vi "Path_Test_TankRobot_ScanIndex.vi"() -> ()   [LabVIEW 2018]
uses:
  Pathfinder-Lib/VIs/Waypoint.ctl
  <vilib>/Rock Robotics/WPI/DriverStation/WPI_DriverStationRobotMode2.ctl
  Pathfinder-Lib/VIs/Wheel_Ctrl_Path_Element.ctl
  Pathfinder-Lib/VIs/Wheel_Ctrl_Path.ctl
  <vilib>/Rock Robotics/SystemInterfaces/AI/FPGA_AIGyroChannel.ctl
  <vilib>/Rock Robotics/SystemInterfaces/DIO/FPGA_DIOChannel.ctl
  <vilib>/Rock Robotics/WPI/Encoder/WPI_EncoderType.ctl
  <vilib>/Rock Robotics/SystemInterfaces/DIO/FPGA_DIOPWMChannel.ctl
  <vilib>/Rock Robotics/WPI/SafetyOutput/WPI_SafetyOutputConfigMenu.ctl
  <vilib>/Rock Robotics/WPI/Gyro/WPI_GyroAnalogOpen.vi
  <vilib>/Rock Robotics/WPI/Counter/WPI_CounterDigitalInputToDigitalSource.vi
  <vilib>/Rock Robotics/WPI/RobotDrive/WPI_RobotDriveOpen2MotorWithTalon.vi
  Robot Global Data.vi
  Secret_Control_Library_Protected/TIME_GET.vi
  <vilib>/addons/control/pid/pid.llb/PID (DBL).vi
  <vilib>/Rock Robotics/Network Tables/NT Write Numeric Array.vi
  <vilib>/Rock Robotics/Network Tables/NT Write Number.vi
  Pathfinder-Lib/Pathfinder.lvlib
  <vilib>/addons/control/pid/NI_PID_pid.lvlib
  Secret_Control_Library_Protected/Secret_Control_Library_Protected.lvlib
panel:
  out "Path \nSpeed > \nMax":bool
  in  "Stop\nProgram":bool
  out "Path Distance":dbl[](array[numeric]) format="%19.2f"
  out "Robot\nExecuting":bool
  in  "Execute\nPath":bool
  out "Ready to \nExecute":bool
  in  "Calculate\nPath":bool
  out "Heading Demand":dbl format="%18.2f"
  out "Gyro Comp":dbl format="%18.2f"
  out "Heading":dbl format="%18.2f"
  in  "Gyro Comp PID gains":T1={"proportional gain (Kc)"=0.065, "integral time (Ti, min)"=0.004, "derivative time (Td, min)"=0.0} {"derivative time (Td, min)" format="%.4f"; "integral time (Ti, min)" format="%.4f"; "proportional gain (Kc)" format="%.4f"}
  out "Path calculation error":errorcluster
  out "Distance":dbl[](array[numeric]) format="%19.2f"
  in  "Use Gyro\nCompensation":bool=TRUE
  out "Heading Error":dbl format="%14.2f"
  out "Distance Error":dbl[](array[numeric]) format="%14.2f"
  out "Robot Mode":T2
  in  "Tab Control":T3(tab)
  in  "max_velocity":dbl=51.5
  in  "max_acceleration":dbl=30.0
  in  "max_jerk":dbl=120.0
  in  "wheelbase_width":dbl=20.866
  out "Real max speed":dbl
  out "Position":cluster{dbl[], dbl[]}[](graph)
  out "Path":T4(graph)
  out "Size":i32
  out "Robot Path Data":T5[](array[typedef]) {"D Time" format="%13.3f"; "Angle" format="%13.3f"; "R dist" format="%13.3f"; "L dist" format="%13.3f"; "R spd" format="%13.3f"; "L spd" format="%13.3f"; "T Time" format="%13.3f"}
  out "Wheel dmd":T6(graph)
  out "Gyro Cht":cluster{"GyroContinuous":dbl, "Angle":dbl}(graph)
  out "Err Chart":cluster{dbl, dbl, dbl}(graph)
  in  "sample_count":i32=1000
  in  "Path Results\ndT":dbl=0.02 format="%7.3f"
  in  "?":T7[](array[typedef])=[{"x"=12.0, "y"=60.0, "angle"=0.0}, {"x"=132.0, "y"=125.0, "angle"=60.0}]
  # "PATH DEFINITION"
  # "ROBOT EXECUTION"
  # "SEC"
  # "Instructions:\nThis should run on a PC simulated robot on or a real robot that has the same motors and sensors.\n1) Enter robot data on Robot Data Tab\n2) Define your path definitions.\n3) Define the time increment.  0.020 is chosen since that matches the normal loop time.\n4) Press calculate path.  If a good path was calculated it will be displayed on the Tank Data tab, and the Ready to Execute will indicate execution can begin.\nThe path can be recalculated many times before selecting execute.\n5) Start the FRC driver station.\n6) Press the execute path button.  This will start the robot simulation, or start running on the roboRIO depending on which target is selected.\n7) On the driver station, select Autonomous Enabled mode to start path execution.\n8) When finished, the graph tabs can be reviwed.  (Usiing the chart tabs during operation breaks the simulation.\n9) When completely done press the Stop Program button to end the programs execution.\n\nNotes:\n- This program alters the left and right motor demands during execution to attempt to match the heading angle demand.  The \nsimulated robot has a lot of drive friction when turning that affects operation.  This example does not include encoder compensation.\nThis could be added.\n- The path generation logic doesn't account distribution of speed to the left and right wheels.  As a result the maximum speed can be exceeded.\nIf this happens, but Path Speed > Max light will light and Ready to Execute will not light.  Lower the maximum speed in the Robot Data tab\nand recalulate the path."
  # "ROBOT DATA"
  # "INCHES/SEC"
  # "INCHES/SEC^2"
  # "?? INCHES/SEC^3"
  # "Simulated robot is 20.866"
  # "INCHES"
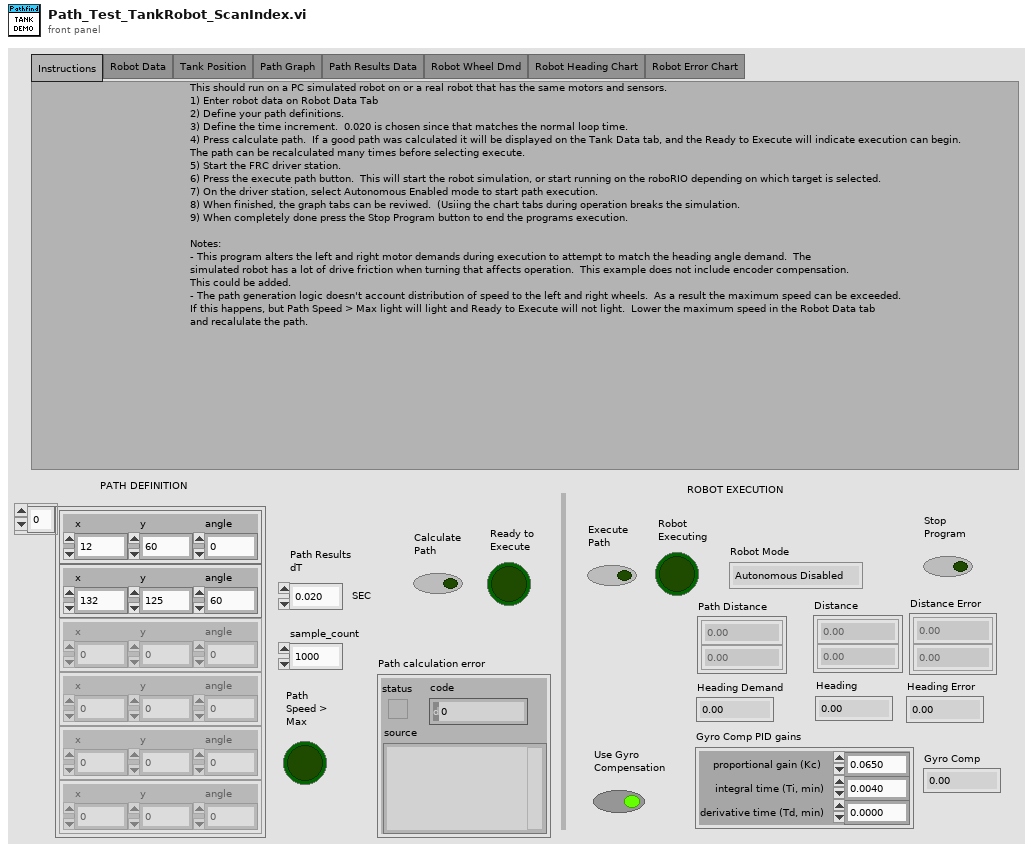
[diagram p1: front panel]
types:
  T1 = cluster{"proportional gain (Kc)":dbl, "integral time (Ti, min)":dbl, "derivative time (Td, min)":dbl}
  T2 = typedef "WPI_DriverStationRobotMode2.ctl" = enum16{"Autonomous Disabled", "Autonomous Enabled", "Teleop Disabled", "Teleop Enabled", "Disconnected", "Finish", "Test Disabled", "Test Enabled", "Emergency Stopped"}
  T3 = enum32{"Instructions", "Robot Data", "Tank Position", "Path Graph", "Path Results Data", "Robot Wheel Dmd", "Robot Heading Chart", "Robot Error Chart"}
  T4 = cluster{"position":dbl, "velocity":dbl, "acceleration":dbl, "jerk":dbl, "heading":dbl}[]
  T5 = typedef "Pathfinder.lvlib/Wheel_Ctrl_Path_Element.ctl" = cluster{"T Time":dbl, "L spd":dbl, "R spd":dbl, "L dist":dbl, "R dist":dbl, "Angle":dbl, "D Time":dbl}
  T6 = cluster{"Output":dbl, "Output":dbl, "output":dbl}
  T7 = typedef "Pathfinder.lvlib/Waypoint.ctl" = cluster{"x":dbl, "y":dbl, "angle":dbl}
  T8 = typedef "Pathfinder.lvlib/Wheel_Ctrl_Path.ctl" = cluster{"Wheel_Ctrl_Elements":T5[], "NumberOfElements":u32, "DeltaMillseconds":i32}
  T9 = typedef "Pathfinder.lvlib/Segment.ctl" = cluster{"dt":dbl, "x":dbl, "y":dbl, "position":dbl, "velocity":dbl, "acceleration":dbl, "jerk":dbl, "heading":dbl}
  T10 = cluster{"position":dbl, "velocity":dbl, "acceleration":dbl, "jerk":dbl, "heading":dbl}
  T11 = typedef "WPI_SafetyOutputConfigMenu.ctl" = enum16{"Enable", "Disable"}
  T12 = typedef "WPI_EncoderType.ctl" = enum16{"1x", "2x", "4x"}
  T13 = typedef "FPGA_AIGyroChannel.ctl" = enum8{"AI 0", "AI 1", "Invalid"}
  T14 = typedef "FPGA_DIOPWMChannel.ctl" = enum8{"PWM 0", "PWM 1", "PWM 2", "PWM 3", "PWM 4", "PWM 5", "PWM 6", "PWM 7", "PWM 8", "PWM 9", "PWM MXP 0", "PWM MXP 1", "PWM MXP 2", "PWM MXP 3", "PWM MXP 4", "PWM MXP 5", "PWM MXP 6", "PWM MXP 7", "PWM MXP 8", "PWM MXP 9", "Invalid"}
  T15 = typedef "FPGA_DIOChannel.ctl" = enum8{"DIO 0", "DIO 1", "DIO 2", "DIO 3", "DIO 4", "DIO 5", "DIO 6", "DIO 7", "DIO 8", "DIO 9", "DIO MXP 0", "DIO MXP 1", "DIO MXP 2", "DIO MXP 3", "DIO MXP 4", "DIO MXP 5", "DIO MXP 6", "DIO MXP 7", "DIO MXP 8", "DIO MXP 9", "DIO MXP 10", "DIO MXP 11", "DIO MXP 12", "DIO MXP 13", "DIO MXP 14", "DIO MXP 15", "SPI Port CS1", "SPI Port CS2", "SPI Port CS3", "SPI Port MISO", "SPI Port MOSI", "Invalid"}
  T16 = typedef "WPI_RobotDriveDevRef.ctl" = cluster{"DevStatus":errorcluster, "Motors[]":T17[], "Square Inputs":bool, "Max Output":dbl}
  T17 = typedef "WPI_MotorControlDeviceRef.ctl" = cluster{"DeviceStatus":errorcluster, "Type":T18, "PWM":cluster{"PWM Channel":T14, "DeadBand":T19}, "CAN":cluster{"Device Number":u8, "SetOutput VI Ref":variant, "GetOutput VI Ref":variant, "Enable VI Ref":variant, "Disable VI Ref":variant, "Data":variant}, "Invert":bool, "DIO PWM":cluster{"PWM \"Enable\" Channel":T14, "DIOChannel":T15, "PWM Rate":dbl}}
  T18 = typedef "WPI_MotorControlType.ctl" = enum16{"PWM", "CAN", "DIO PWM"}
  T19 = typedef "WPI_PWMDeadband.ctl" = cluster{"Name":string, "maxPositivePwm":i32, "minPositivePwm":i32, "centerPwm":i32, "maxNegativePwm":i32, "minNegativePwm":i32, "angularRange":u16}
  T20 = typedef "WPI_DigitalInputDevRef.ctl" = cluster{"DevStatus":errorcluster, "DIO Channel":T15}
  T21 = typedef "FPGA_CounterEncoderSourceConvertionLVSourceType.ctl" = cluster{"DevStatus":errorcluster, "AnalogTriggerMode?":bool, "DigitalMode":cluster{"DIO Channel":T22}, "AnalogTriggerMode":cluster{"AnalogTriggerIndex":T23, "OutputType":T24}}
  T22 = typedef "FPGA_DIODigitalSourceChannel.ctl" = enum8{"DIO 0", "DIO 1", "DIO 2", "DIO 3", "DIO 4", "DIO 5", "DIO 6", "DIO 7", "DIO 8", "DIO 9", "DIO MXP 0", "DIO MXP 1", "DIO MXP 2", "DIO MXP 3", "DIO MXP 4", "DIO MXP 5", "DIO MXP 6", "DIO MXP 7", "DIO MXP 8", "DIO MXP 9", "DIO MXP 10", "DIO MXP 11", "DIO MXP 12", "DIO MXP 13", "DIO MXP 14", "DIO MXP 15", "SPI Port CS1", "SPI Port CS2", "SPI Port CS3", "SPI Port MISO", "SPI Port MOSI", "Disabled"}
  T23 = typedef "FPGA_AnalogTriggerIndex.ctl" = enum8{"Trig 0", "Trig 1", "Trig 2", "Trig 3", "Trig 4", "Trig 5", "Trig 6", "Trig 7", "Invalid"}
  T24 = typedef "FPGA_AnalogTriggerOutType.ctl" = enum16{"InWindow", "TriggerState", "Rising", "Falling"}
  T25 = typedef "WPI_EncoderDevRef.ctl" = cluster{"DevStatus":errorcluster, "EncoderIndex":T26, "CounterIndex":T27, "DistancePerCount":dbl, "Decoding Type":T12}
  T26 = typedef "FPGA_EncoderIdx.ctl" = enum8{"Enc 0", "Enc 1", "Enc 2", "Enc 3", "Enc 4", "Enc 5", "Enc 6", "Enc 7", "Invalid"}
  T27 = typedef "FPGA_CounterCtrSystemIndex.ctl" = enum8{"Ctr 0", "Ctr 1", "Ctr 2", "Ctr 3", "Ctr 4", "Ctr 5", "Ctr 6", "Ctr 7", "Invalid"}
  T28 = typedef "WPI_GyroDevRef.ctl" = cluster{"DevStatus":errorcluster, "Analog Channel":T29, "Gain (VoltsPerDegree/Second)":dbl, "Gyro Type":enum16{"Analog", "XRS450"}, "Handle":i32, "SPI Bus":T30, "Device Found":bool, "Sample Rate":dbl, "Calibrate On Open":bool, "Offset":dbl}
  T29 = typedef "FPGA_AIChannel.ctl" = enum8{"AI 0", "AI 1", "AI 2", "AI 3", "AI MXP 0", "AI MXP 1", "AI MXP 2", "AI MXP 3", "Invalid"}
  T30 = typedef "spi_bus.ctl" = enum16{"SPI On-Board, CS0", "SPI On-Board, CS1", "SPI On-Board, CS2", "SPI On-Board, CS3", "SPI MXP", "Invalid"}
  T31 = cluster{"GyroContinuous":dbl, "GyroContinuous":dbl}
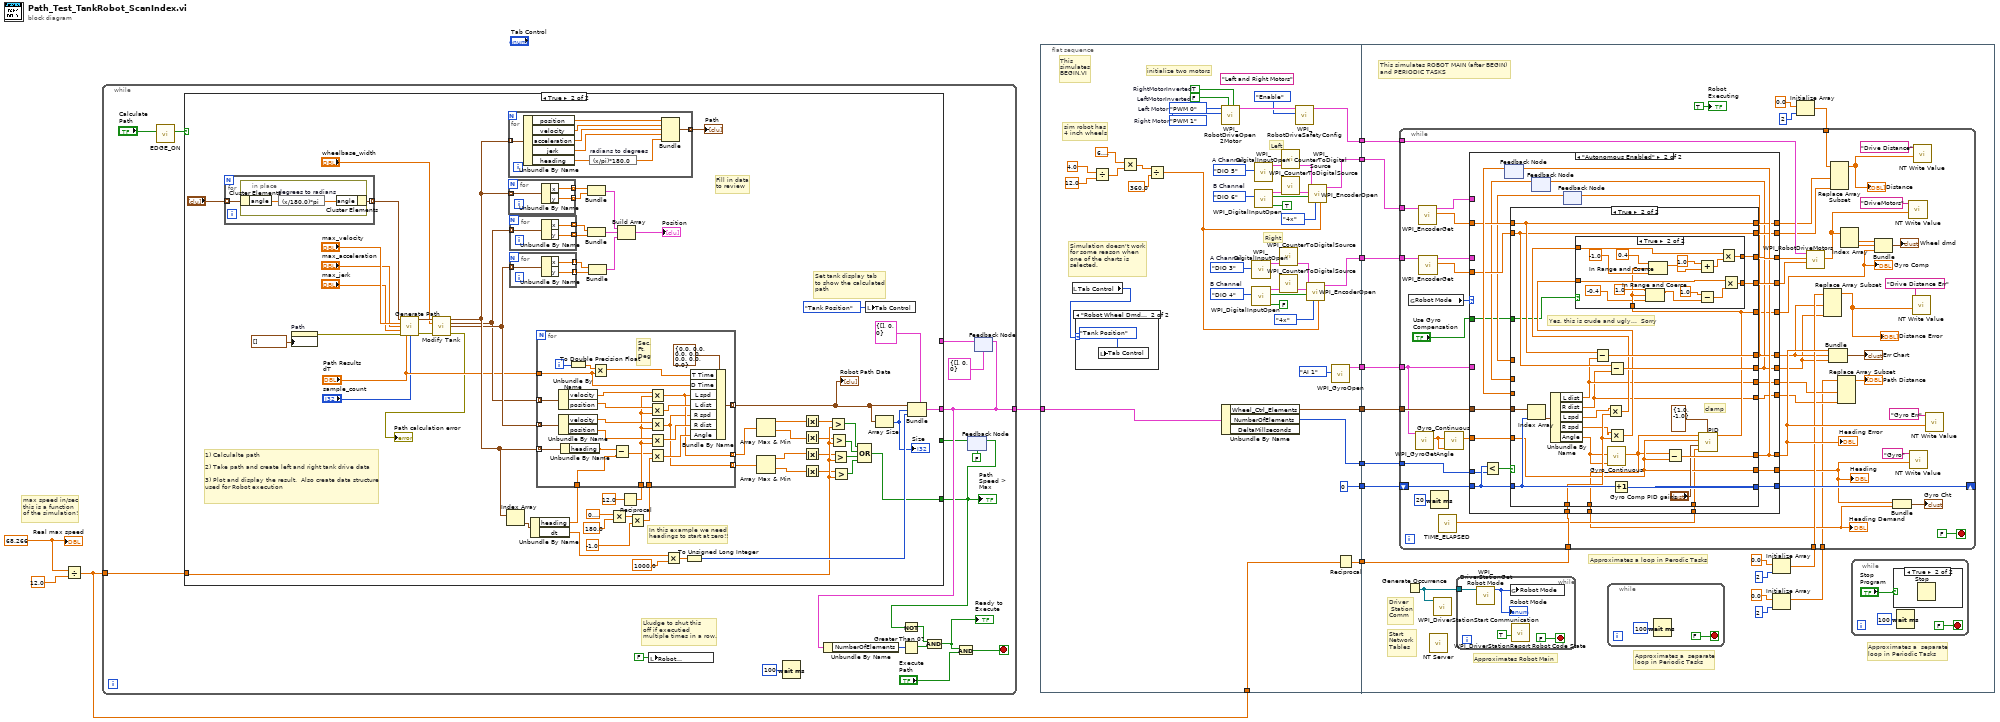
[diagram p0: block diagram]
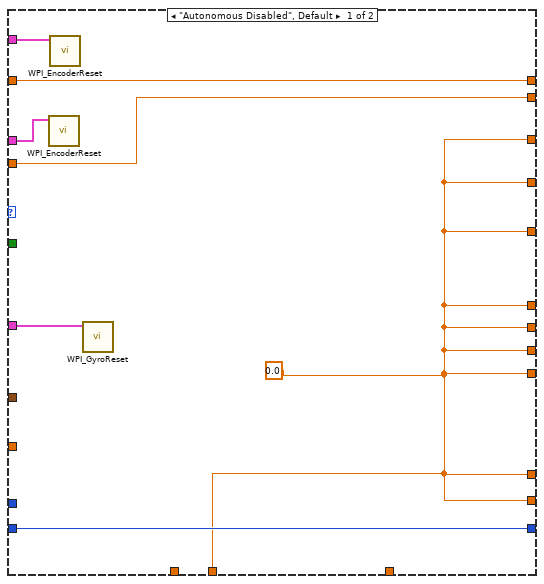
[diagram p5: hidden frame]
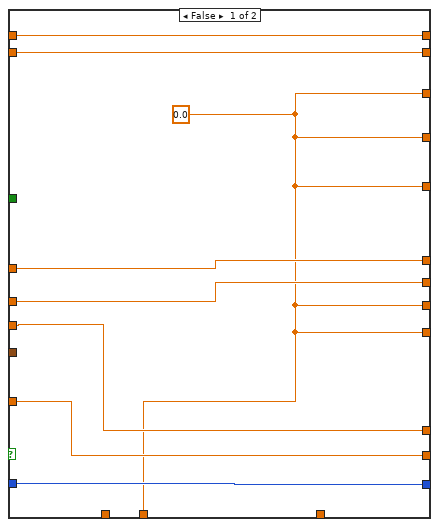
[diagram p6: hidden frame]
diagram:
  w3 = 68.266 ("x")
  # "max speed in/sec\nthis is a function\nof the simulation!"
  n1 = Divide(x=w3, y=12.0) -> (x/y=w2:dbl)
  n2 = while {
    tunnel: [w24] -> w12
    tunnel: w2 -> [w19]
    stop <- w21 stop-if-true
    # "Lkudge to shut this\noff if executied\nmultiple times in a row."
    n3 = call "EDGE_ON.vi"("INPUT"="Calculate\nPath") -> ("EDGE ON"=w27:bool)  [unwired: 10 in]
    n4 = local write "Robot\nExecuting"(FALSE ("Robot\nExecuting")) -> ()
    n5 = Wait (ms)(milliseconds to wait=u32 100) -> ()  [unwired: 1 out]
    n6 = feedback #1(FALSE) -> (w17:bool)
    n7 = feedback #2(T8 {"Wheel_Ctrl_Elements"=[], "NumberOfElements"=0, "DeltaMillseconds"=0} ("Wheel_Ctrl_Elements")) -> (w25:T8)
    n8 = case shown="True" w27 {
      tunnel: [w31 w51] -> w24
      tunnel: w25 -> [w31 _]
      tunnel: w19 -> [_ w49]
      tunnel: [w30 w40] -> w13
      tunnel: w17 -> [w30 _]
      frame False {
      }
      frame True {
        # "Set tank display tab\nto show the calculated\npath"
        # "Fill in data\nto review"
        # "1) Calculalte path\n\n2) Take path and create left and right tank drive data\n\n3) Plot and display the result.  Also create data structure\nused for Robot execution"
        # "In this example we need\nheadings to start at zero!!"
        n9 = for {
          tunnel: "?" -> [w117] mode=indexing
          tunnel: [w116] -> w77 mode=indexing
          n10 = in-place {
            n11 = in-place-cluster #3(w117) -> ("angle"=w119:dbl)
            n12 = expression code="(x/180.0)*pi" "degrees to radians"(w119) -> (w118:dbl)
            n13 = in-place-cluster #3("angle"=w118) -> (w116:T7)
          }
        }
        n14 = property on="Path" class="WFChart (strict)"("History Data"=T4 []) -> (error out=w79:errorcluster)  [unwired: 2 in, 1 out]
        n15 = call "Generate Path.vi"("path"=w77, "max_velocity"="max_velocity", "max_acceleration"="max_acceleration", "max_jerk"="max_jerk", "error in"=w79, "dt (.001)"="Path Results\ndT", "sample_count (100000)"="sample_count") -> ("Segments"=w80:T9[], "error out"=w66:errorcluster)  [unwired: 7 in]
        n16 = call "Modify Tank.vi"("Original"=w80, "wheelbase_width"="wheelbase_width", "error in"=w66) -> ("original"=w90:T9[], "left"=w85:T9[], "right"=w86:T9[], "error out"=→"Path calculation error":errorcluster)  [unwired: 9 in]
        n17 = Index Array(array=w90) -> (element=w91:T9)  [unwired: 1 in]
        n18 = for {
          tunnel: w90 -> [w136] mode=indexing
          tunnel: [w130] -> w82 mode=indexing
          n19 = Unbundle By Name(w136) -> ("position"=w135:dbl, "velocity"=w134:dbl, "acceleration"=w133:dbl, "jerk"=w132:dbl, "heading"=w131:dbl)
          n20 = expression code="(x/pi)*180.0" "radians to degrees"(w131) -> (w129:dbl)
          n21 = Bundle("position"=w135, "velocity"=w134, "acceleration"=w133, "jerk"=w132, "heading"=w129) -> (w130:T10)  [unwired: 1 in]
        }
        "Path" <- w82
        n22 = for {
          tunnel: w90 -> [w122] mode=indexing
          tunnel: [w121] -> w74 mode=indexing
          tunnel: [w120] -> w75 mode=indexing
          n23 = Unbundle By Name(w122) -> ("x"=w121:dbl, "y"=w120:dbl)
        }
        n24 = for {
          tunnel: w85 -> [w128] mode=indexing
          tunnel: [w127] -> w68 mode=indexing
          tunnel: [w126] -> w69 mode=indexing
          n25 = Unbundle By Name(w128) -> ("x"=w127:dbl, "y"=w126:dbl)
        }
        n26 = for {
          tunnel: w86 -> [w125] mode=indexing
          tunnel: [w124] -> w70 mode=indexing
          tunnel: [w123] -> w71 mode=indexing
          n27 = Unbundle By Name(w125) -> ("x"=w124:dbl, "y"=w123:dbl)
        }
        n28 = Unbundle By Name(w91) -> ("heading"=w92:dbl, "dt"=w55:dbl)
        n29 = Bundle(w74, w75) -> (w76:cluster{dbl[], dbl[]})  [unwired: 1 in]
        n30 = Bundle(w68, w69) -> (w73:cluster{dbl[], dbl[]})  [unwired: 1 in]
        n31 = Bundle(w70, w71) -> (w72:cluster{dbl[], dbl[]})  [unwired: 1 in]
        n32 = Multiply(x=0.3183098861837907, y=180.0) -> (x*y=w88:dbl)
        n33 = Build Array(w76, w73, w72) -> (→"Position":cluster{dbl[], dbl[]}[])
        n34 = Reciprocal(x=12.0) -> (1/x=w84:dbl)
        n35 = Multiply(x=w88, y=-1.0) -> (x*y=w89:dbl)
        n36 = for {
          tunnel: "Path Results\ndT" -> [w111]
          tunnel: [w114] -> w39 mode=indexing
          tunnel: w84 -> [w106]
          tunnel: w89 -> [w105]
          tunnel: w85 -> [w101] mode=indexing
          tunnel: w86 -> [w100] mode=indexing
          tunnel: w90 -> [w99] mode=indexing
          tunnel: w92 -> [w96]
          tunnel: [w94] -> w38 mode=indexing
          tunnel: [w93] -> w37 mode=indexing
          i -> [w113]
          # "Sec,\nFt,\nDeg"
          n37 = Unbundle By Name(w101) -> ("velocity"=w110:dbl, "position"=w109:dbl)
          n38 = Unbundle By Name(w100) -> ("velocity"=w108:dbl, "position"=w107:dbl)
          n39 = Unbundle By Name(w99) -> ("heading"=w97:dbl)
          n40 = To Double Precision Float(number=w113) -> (double precision float=w115:dbl)
          n41 = Multiply(x=w115, y=w111) -> (x*y=w112:dbl)
          n42 = Subtract(x=w97, y=w96) -> (x-y=w98:dbl)
          n43 = Multiply(x=w110, y=w106) -> (x*y=w94:dbl)
          n44 = Multiply(x=w109, y=w106) -> (x*y=w104:dbl)
          n45 = Multiply(x=w108, y=w106) -> (x*y=w93:dbl)
          n46 = Multiply(x=w107, y=w106) -> (x*y=w103:dbl)
          n47 = Multiply(x=w98, y=w105) -> (x*y=w102:dbl)
          n48 = Bundle By Name(cluster=T5 {"T Time"=0.0, "L spd"=0.0, "R spd"=0.0, "L dist"=0.0, "R dist"=0.0, "Angle"=0.0, "D Time"=0.0} ("Wheel dmd"), "T Time"=w112, "D Time"=w111, "L spd"=w94, "L dist"=w104, "R spd"=w93, "R dist"=w103, "Angle"=w102) -> (w114:T5)
        }
        "Robot Path Data" <- w39
        n49 = Multiply(x=w55, y=1000.0) -> (x*y=w53:dbl)
        n50 = To Unsigned Long Integer(number=w53) -> (unsigned 32bit integer=w52:u32)
        n51 = Array Max & Min(array=w38) -> (max value=w36:dbl, min value=w35:dbl)  [unwired: 2 out]
        n52 = Array Max & Min(array=w37) -> (max value=w34:dbl, min value=w33:dbl)  [unwired: 2 out]
        n53 = Absolute Value(x=w36) -> (abs(x)=w48:dbl)
        n54 = Absolute Value(x=w35) -> (abs(x)=w47:dbl)
        n55 = Absolute Value(x=w34) -> (abs(x)=w46:dbl)
        n56 = Absolute Value(x=w33) -> (abs(x)=w45:dbl)
        n57 = Greater?(x=w48, y=w49) -> (0:w44:bool)
        n58 = Greater?(x=w47, y=w49) -> (0:w43:bool)
        n59 = Greater?(x=w46, y=w49) -> (0:w42:bool)
        n60 = Greater?(x=w45, y=w49) -> (0:w41:bool)
        n61 = Compound Arithmetic op=OR(w44, w43, w42, w41) -> (w40:bool)
        n62 = local write "Tab Control"(T3."Tank Position" ("Tab Control")) -> ()
        n63 = Array Size(array=w39) -> (size(s)=w50:i32)
        "Size" <- w50
        n64 = Bundle(cluster=T8 {"Wheel_Ctrl_Elements"=[], "NumberOfElements"=0, "DeltaMillseconds"=0} ("Wheel_Ctrl_Elements"), "Wheel_Ctrl_Elements"=w39, "NumberOfElements"=w50, "DeltaMillseconds"=w52) -> (w51:T8)
      }
    }
    "Path \nSpeed > \nMax" <- w13
    n65 = Unbundle By Name(w24) -> ("NumberOfElements"=w23:u32)
    n66 = Not(x=w13) -> (.not. x?=w15:bool)
    n67 = Greater Than 0?(x=w23) -> (x > 0?=w16:bool)
    n68 = And(x=w15, y=w16) -> (x .and. y?=w14:bool)
    "Ready to \nExecute" <- w14
    n69 = And(x=w14, y="Execute\nPath") -> (x .and. y?=w21:bool)
    n70 = feedback-in #1(w13) -> ()
    n71 = feedback-in #2(w24) -> ()
  }
  n72 = flat-sequence {
    tunnel: w12 -> [w143]
    tunnel: [w146] -> w11
    tunnel: [w176] -> w10
    tunnel: [w144] -> w9
    tunnel: [w145] -> w8
    tunnel: [w142] -> w7
    tunnel: [w141] -> w6
    tunnel: [w140] -> w5
    tunnel: w2 -> [w139]
    tunnel: [0] -> w1
    tunnel: w11 -> [w195]
    tunnel: w10 -> [w194]
    tunnel: w9 -> [w193]
    tunnel: w8 -> [w186]
    tunnel: w7 -> [w196]
    tunnel: w6 -> [w185]
    tunnel: w5 -> [w180]
    tunnel: w1 -> [w179]
    frame #0 {
      w160 = FPGA_DIOPWMChannel."PWM 1"  # Right Motor
      w159 = FPGA_DIOPWMChannel."PWM 0"  # Left Motor
      (unwired) "Left and Right Motors" ("refnum name")
      w161 = FALSE  # LeftMotorInverted
      w162 = TRUE  # RightMotorInverted
      w154 = FPGA_DIOChannel."DIO 4"  # B Channel
      w153 = FPGA_DIOChannel."DIO 3"  # A Channel
      w150 = FPGA_DIOChannel."DIO 6"  # B Channel
      w149 = FPGA_DIOChannel."DIO 5"  # A Channel
      # "Simulation doesn't work\nfor some reason when\none of the charts is\nselected."
      # "This \nsimulates\nBEGIN.VI"
      # "sim robot has\n4 inch wheels"
      # "initialize two motors"
      # "Right"
      # "Left"
      n73 = local read "Tab Control"() -> (w137:T3)
      n74 = case shown="\"Robot Wheel Dmd\"..\"Robot Error Chart\"" w137 {
        frame Default {
        }
        frame "Robot Wheel Dmd".."Robot Error Chart" {
          n75 = local write "Tab Control"(T3."Tank Position" ("Tab Control")) -> ()
        }
      }
      n76 = Divide(x=4.0, y=12.0) -> (x/y=w172:dbl)
      n77 = Multiply(x=6.283185307179586, y=w172) -> (x*y=w173:dbl)
      n78 = Divide(x=w173, y=360.0) -> (x/y=w174:dbl)
      n79 = call-poly <vilib>:"WPI_RobotDriveOpen2Motor.vi"("Right Motor Inverted"=w162, "Left Motor Inverted"=w161, "Right Motor"=w160, "Left Motor"=w159) -> ("RobotDriveDevRef"=w175:T16)  [unwired: 1 in, 6 out]
      n80 = Unbundle By Name(w143) -> ("Wheel_Ctrl_Elements"=w142:T5[], "NumberOfElements"=w141:u32)  [unwired: 1 out]
      n81 = call <vilib>:"WPI_DigitalInputOpen.vi"("DIO Channel"=w153) -> ("DigitalInputDevRef"=w170:T20)  [unwired: 1 in, 9 out]
      n82 = call <vilib>:"WPI_DigitalInputOpen.vi"("DIO Channel"=w154) -> ("DigitalInputDevRef"=w169:T20)  [unwired: 1 in, 9 out]
      n83 = call <vilib>:"WPI_DigitalInputOpen.vi"("DIO Channel"=w149) -> ("DigitalInputDevRef"=w166:T20)  [unwired: 1 in, 9 out]
      n84 = call <vilib>:"WPI_DigitalInputOpen.vi"("DIO Channel"=w150) -> ("DigitalInputDevRef"=w165:T20)  [unwired: 1 in, 9 out]
      n85 = call-poly <vilib>:"WPI_CounterToDigitalSource.vi"("DigitalInputDevRef"=w170) -> ("Digital Source"=w171:T21)  [unwired: 6 out]
      n86 = call-poly <vilib>:"WPI_CounterToDigitalSource.vi"("DigitalInputDevRef"=w169) -> ("Digital Source"=w168:T21)  [unwired: 6 out]
      n87 = call-poly <vilib>:"WPI_CounterToDigitalSource.vi"("DigitalInputDevRef"=w166) -> ("Digital Source"=w167:T21)  [unwired: 6 out]
      n88 = call-poly <vilib>:"WPI_CounterToDigitalSource.vi"("DigitalInputDevRef"=w165) -> ("Digital Source"=w164:T21)  [unwired: 6 out]
      n89 = call <vilib>:"WPI_RobotDriveSafetyConfig.vi"("mode"=WPI_SafetyOutputConfigMenu."Enable", "RobotDriveDevRef"=w175) -> ("RobotDriveDevRef"=w146:T16)  [unwired: 8 in, 1 out]
      n90 = call <vilib>:"WPI_EncoderOpen.vi"("DistancePerCount"=w174, "Decoding Type"=WPI_EncoderType."4x", "Invert Direction (False)"=FALSE, "BSource"=w168, "ASource"=w171) -> ("EncoderDevRef"=w145:T25)  [unwired: 3 in, 3 out]
      n91 = call <vilib>:"WPI_EncoderOpen.vi"("DistancePerCount"=w174, "Decoding Type"=WPI_EncoderType."4x", "Invert Direction (False)"=TRUE, "BSource"=w164, "ASource"=w167) -> ("EncoderDevRef"=w144:T25)  [unwired: 3 in, 3 out]
      n92 = call-poly <vilib>:"WPI_GyroOpen.vi"("Analog Channel"=FPGA_AIGyroChannel."AI 1") -> ("GyroDevRef"=w176:T28)  [unwired: 8 in, 2 out]
      n93 = Reciprocal(x=w139) -> (1/x=w140:dbl)
    }
    frame #1 {
      # "Approximates a  separate\nloop in Periodic Tasks"
      # "This simulates ROBOT MAIN (after BEGIN)\nand PERIODIC TASKS"
      # "Approximates a loop in Perodic Tasks"
      # "Approximates a  separate\nloop in Periodic Tasks"
      # "Approximates Robot Main"
      # "Start\nNetwork\nTables"
      # "Driver\n Station\nComm"
      n94 = Generate Occurrence() -> (w197:refnum<k4>)
      n95 = call <vilib>:"NT Server.vi"() -> ()  [unwired: 12 in]
      n96 = call <vilib>:"WPI_DriverStationStart Communication.vi"("occurrence"=w197) -> ()  [unwired: 11 in]
      n97 = while {
        tunnel: w197 -> [w339]
        stop <- FALSE stop-if-true
        n98 = call <vilib>:"WPI_DriverStationGet Robot Mode.vi"("DS Occurrence"=w339) -> ("Robot Mode"=w336:T2)  [unwired: 1 in, 9 out]
        "Robot Mode" <- w336
        n99 = global write "Robot Global Data.vi" "Robot Mode"(w336) -> ()
        n100 = call <vilib>:"WPI_DriverStationReport Robot Code State.vi"("TeleOp"=TRUE ("Autonomous")) -> ()  [unwired: 10 in, 1 out]
      }
      n101 = while {
        stop <- FALSE stop-if-true
        n102 = Wait (ms)(milliseconds to wait=u32 100) -> ()  [unwired: 1 out]
      }
      n103 = Initialize Array(0.0, 2 ("dimension size")) -> (w187:dbl[])
      n104 = Initialize Array(0.0, 2 ("dimension size")) -> (w181:dbl[])
      n105 = Initialize Array(0.0, 2 ("dimension size")) -> (w190:dbl[])
      n106 = while {
        tunnel: w196 -> [w242]
        tunnel: w195 -> [w247]
        shift-right: [w243] -> _
        shift-left: w179 -> [w244]
        tunnel: w194 -> [w239]
        tunnel: w193 -> [w237]
        tunnel: w180 -> [w231]
        tunnel: w190 -> [w227]
        tunnel: w187 -> [w223]
        tunnel: w186 -> [w207]
        tunnel: w185 -> [w206]
        tunnel: w181 -> [w202]
        stop <- FALSE stop-if-true
        n107 = global read "Robot Global Data.vi" "Robot Mode"() -> (w248:T2)
        n108 = call <vilib>:"WPI_GyroGetAngle.vi"("GyroDevRef"=w239) -> ("Angle"=w213:dbl)  [unwired: 7 in, 3 out]
        n109 = call <vilib>:"WPI_EncoderGet.vi"("EncoderDevRef"=w237) -> ("Distance"=w234:dbl, "EncoderDevRef"=w208:T25)  [unwired: 5 in, 4 out]
        n110 = call <vilib>:"WPI_EncoderGet.vi"("EncoderDevRef"=w207) -> ("Distance"=w233:dbl, "EncoderDevRef"=w236:T25)  [unwired: 5 in, 4 out]
        n111 = Wait (ms)(milliseconds to wait=u32 20) -> ()  [unwired: 1 out]
        n112 = call "TIME_ELAPSED.vi"() -> ("Elapsed Sec"=w212:dbl)  [unwired: 11 in]
        n113 = call "Gyro_Continuous.vi"("GyroInitial"=w213, "GyroInput"=w213) -> ("GyroContinuous"=w219:dbl)  [unwired: 9 in]
        n114 = case shown="\"Autonomous Enabled\"" w248 {
          tunnel: [w250 w279] -> w246
          tunnel: [w250 w280] -> w245
          tunnel: w244 -> [w256 w282]
          tunnel: [w256 w281] -> w243
          tunnel: w242 -> [_ w278]
          tunnel: w231 -> [_ w276]
          tunnel: w239 -> [w255 _]
          tunnel: w219 -> [_ w275]
          tunnel: [w250 w274] -> w210
          tunnel: [w250 w273] -> w229
          tunnel: w236 -> [w254 _]
          tunnel: w234 -> [w253 w271]
          tunnel: w233 -> [w252 w270]
          tunnel: [w253 w269] -> w226
          tunnel: [w252 w268] -> w225
          tunnel: [w250 w264] -> w220
          tunnel: [w250 w265] -> w221
          tunnel: "Use Gyro\nCompensation" -> [_ w263]
          tunnel: [w250 w262] -> w215
          tunnel: w212 -> [_ w261]
          tunnel: [w250 w260] -> w209
          tunnel: w208 -> [w251 _]
          tunnel: w206 -> [_ w259]
          tunnel: [w250 w258] -> w204
          tunnel: [w250 w257] -> w203
          frame "Autonomous Disabled", Default {
            w250 = 0.0
            n115 = call <vilib>:"WPI_EncoderReset.vi"("EncoderDevRef"=w254) -> ()  [unwired: 9 in, 2 out]
            n116 = call <vilib>:"WPI_EncoderReset.vi"("EncoderDevRef"=w251) -> ()  [unwired: 9 in, 2 out]
            n117 = call <vilib>:"WPI_GyroReset.vi"("GyroDevRef"=w255) -> ()  [unwired: 9 in, 2 out]
          }
          frame "Autonomous Enabled" {
            n118 = Less?(x=w282, y=w259) -> (x < y?=w277:bool)
            n119 = feedback #4() -> (w272:dbl)  [unwired: 1 in]
            n120 = feedback #5() -> (w266:dbl)  [unwired: 1 in]
            n121 = feedback #6() -> (w267:dbl)  [unwired: 1 in]
            n122 = case shown="True" w277 {
              tunnel: w282 -> [w290 w315]
              tunnel: [w290 w316] -> w281
              tunnel: [w283 w313] -> w280
              tunnel: [w283 w312] -> w279
              tunnel: w278 -> [_ w296]
              tunnel: w276 -> [_ w314]
              tunnel: w275 -> [w289 w300]
              tunnel: [w289 w300] -> w274
              tunnel: [w288 w304] -> w273
              tunnel: w272 -> [w288 _]
              tunnel: w271 -> [w286 w311]
              tunnel: [w286 w311] -> w269
              tunnel: w270 -> [w287 w310]
              tunnel: [w287 w310] -> w268
              tunnel: w267 -> [w285 _]
              tunnel: w266 -> [w284 _]
              tunnel: [w284 w309] -> w264
              tunnel: [w285 w308] -> w265
              tunnel: w263 -> [_ w305]
              tunnel: [w283 w301] -> w262
              tunnel: w261 -> [_ w299]
              tunnel: [w283 w298] -> w260
              tunnel: [w283 w292] -> w258
              tunnel: [w283 w291] -> w257
              frame False {
                w283 = 0.0
              }
              frame True {
                # "Yes, this is crude and ugly...  Sorry"
                # "clamp"
                n123 = Index Array(array=w296, index=w315) -> (element=w294:T5)
                n124 = Unbundle By Name(w294) -> ("L dist"=w292:dbl, "R dist"=w291:dbl, "L spd"=w297:dbl, "R spd"=w293:dbl, "Angle"=w295:dbl)
                n125 = Subtract(x=w311, y=w292) -> (x-y=w308:dbl)
                n126 = Multiply(x=w297, y=w314) -> (x*y=w307:dbl)
                n127 = Subtract(x=w310, y=w291) -> (x-y=w309:dbl)
                n128 = Multiply(x=w293, y=w314) -> (x*y=w306:dbl)
                n129 = call "Gyro_Continuous.vi"("GyroInitial"=w295, "GyroInput"=w295) -> ("GyroContinuous"=w298:dbl)  [unwired: 9 in]
                n130 = Increment(x=w315) -> (x+1=w316:i32)
                n131 = Subtract(x=w298, y=w300) -> (x-y=w304:dbl)
                n132 = call-poly <vilib>:"PID.vi"("output range"=cluster{"output high":dbl, "output low":dbl} {"output high"=1.0, "output low"=-1.0}, "dt (s)"=w299, "PID gains"="Gyro Comp PID gains", "process variable"=w300, "setpoint"=w298) -> ("output"=w301:dbl)  [unwired: 5 in, 1 out]
                n133 = case shown="True" w305 {
                  tunnel: [w317 w329] -> w313
                  tunnel: w307 -> [w318 w328]
                  tunnel: [w318 w327] -> w312
                  tunnel: w306 -> [w317 w326]
                  tunnel: w301 -> [_ w320]
                  frame False {
                  }
                  frame True {
                    n134 = In Range and Coerce(upper limit=1.0, x=w320, lower limit=-0.4 ("x")) -> (coerced(x)=w322:dbl)  [unwired: 1 out]
                    n135 = In Range and Coerce(upper limit=0.4, x=w320, lower limit=-1.0 ("x")) -> (coerced(x)=w323:dbl)  [unwired: 1 out]
                    n136 = Add(x=1.0, y=w323) -> (x+y=w332:dbl)
                    n137 = Subtract(x=1.0, y=w322) -> (x-y=w330:dbl)
                    n138 = Multiply(x=w328, y=w332) -> (x*y=w327:dbl)
                    n139 = Multiply(x=w326, y=w330) -> (x*y=w329:dbl)
                  }
                }
              }
            }
            n140 = feedback-in #4(w273) -> ()
            n141 = feedback-in #5(w264) -> ()
            n142 = feedback-in #6(w265) -> ()
          }
        }
        "Heading Error" <- w229
        "Heading" <- w210
        "Gyro Comp" <- w215
        "Heading Demand" <- w209
        n143 = call <vilib>:"WPI_RobotDriveMotors.vi"("RightSpeed"=w245, "LeftSpeed"=w246, "RobotDriveDevRef"=w247) -> ("Motor Values"=w218:dbl[])  [unwired: 6 in, 2 out]
        n144 = Replace Array Subset(array=w223, new element #1=w221, new element #2=w220) -> (w222:dbl[])  [unwired: 2 in]
        "Distance Error" <- w222
        n145 = Bundle(w229, w221, w220) -> (→"Err Chart":cluster{dbl, dbl, dbl})  [unwired: 1 in]
        n146 = Replace Array Subset(array=w227, new element #1=w226, new element #2=w225) -> (w224:dbl[])  [unwired: 2 in]
        "Distance" <- w224
        n147 = Replace Array Subset(array=w202, new element #1=w204, new element #2=w203) -> (→"Path Distance":dbl[])  [unwired: 2 in]
        n148 = Index Array(array=w218) -> (element #1=w216:dbl, element #2=w217:dbl)  [unwired: 2 in]
        n149 = Bundle("Output"=w216, "Output"=w217, "output"=w215) -> (→"Wheel dmd":T6)  [unwired: 1 in]
        n150 = Bundle("GyroContinuous"=w210, "GyroContinuous"=w209) -> (→"Gyro Cht":T31)  [unwired: 1 in]
        n151 = call-poly <vilib>:"NT Write Value.vi"("Numeric Array"=w218, "Name"="DriveMotors") -> ()  [unwired: 9 in, 1 out]
        n152 = call-poly <vilib>:"NT Write Value.vi"("Numeric"=w210, "Name"="Gyro") -> ()  [unwired: 9 in, 1 out]
        n153 = call-poly <vilib>:"NT Write Value.vi"("Numeric Array"=w222, "Name"="Drive Distance Err") -> ()  [unwired: 9 in, 1 out]
        n154 = call-poly <vilib>:"NT Write Value.vi"("Numeric Array"=w224, "Name"="Drive Distance") -> ()  [unwired: 9 in, 1 out]
        n155 = call-poly <vilib>:"NT Write Value.vi"("Numeric"=w229, "Name"="Gyro Err") -> ()  [unwired: 9 in, 1 out]
      }
      n156 = while {
        stop <- FALSE stop-if-true
        n157 = case shown="True" "Stop\nProgram" {
          frame False {
          }
          frame True {
            n158 = Stop() -> ()  [unwired: 1 in]
          }
        }
        n159 = Wait (ms)(milliseconds to wait=u32 100) -> ()  [unwired: 1 out]
      }
      "Robot\nExecuting" <- TRUE ("Robot\nExecuting")
    }
  }
  "Real max speed" <- w3
